vi "atcs_logEvent_SpectrographInPosition.vi"(8 "error in (no error)":errorcluster, 11 "logevent_SpectrographInPosition_Ctl":T1) -> (0 "error out":errorcluster, 2 "function return":i32, 3 "logevent_SpectrographInPosition_Ctl out":T1)   [LabVIEW 2016, in "SALLV_atcs.lvlib"]
doc: "int atcs_shm_logEvent_SpectrographInPositionLV(atcs_logevent_SpectrographInPositionLV *logevent_SpectrographInPosition_Ctl );"
uses:
  SALLV_atcs.lvlib
  DataTypes/logevent_SpectrographInPosition.ctl
  SALLV_atcs.so
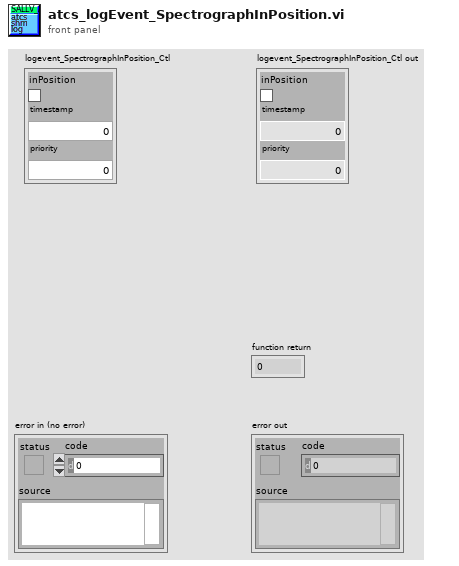
[diagram p1: front panel]
types:
  T1 = typedef "SALLV_atcs.lvlib/logevent_SpectrographInPosition.ctl" = cluster{"inPosition":bool, "timestamp":dbl, "priority":i32}
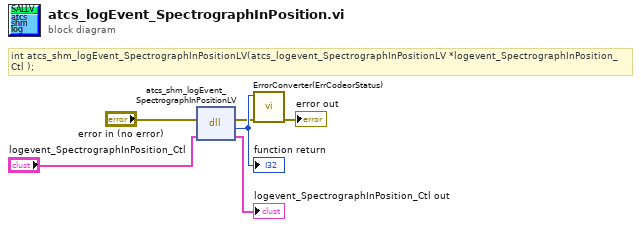
[diagram p0: block diagram]
diagram:
  # "int atcs_shm_logEvent_SpectrographInPositionLV(atcs_logevent_SpectrographInPositionLV *logevent_SpectrographInPosition_Ctl );"
  n1 = dll-call lib="home/andres/Desktop/SALLV_atcs/SALLV_atcs.*" fn="atcs_shm_logEvent_SpectrographInPositionLV"(error in="error in (no error)", "logevent_SpectrographInPosition_Ctl"="logevent_SpectrographInPosition_Ctl") -> (error out=w2:errorcluster, w6:i32, "logevent_SpectrographInPosition_Ctl"=→"logevent_SpectrographInPosition_Ctl out":T1)  [unwired: 2 in, 1 out]
  "function return" <- w6
  n2 = call "ErrorConverter(ErrCodeorStatus).vi"("error in (no error)"=w2, "error code"=w6) -> ("error out"=→"error out":errorcluster)  [unwired: 9 in]
